vi "S2C_SetXmlOutput.vi"(8 "Error In":errorcluster, 11 "MenuRef":refnum<k9>) -> (0 "Error Out":errorcluster)   [LabVIEW 2015]
doc: "Toggles the \"Local File\" runtime menu item."
uses:
  XML/S2C_XML_Globals.vi
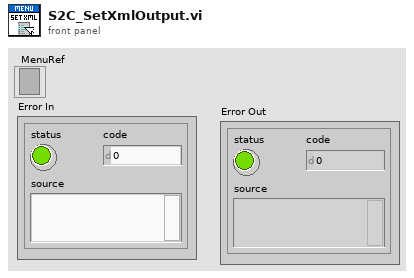
[diagram p1: front panel]
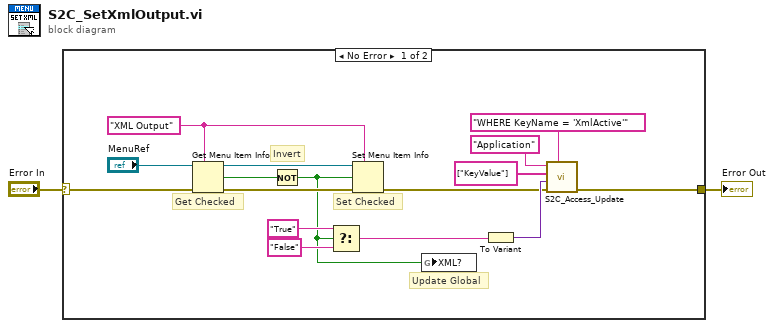
[diagram p0: block diagram]
diagram:
  n1 = case shown="No Error" "Error In" {
    selector: "Error In" -> [w18 w19]
    tunnel: [w5 w19] -> w1
    frame No Error {
      w16 = "XML Output" ("item tag")
      # "Update Global"
      # "Invert"
      # "Set Checked"
      # "Get Checked"
      n2 = Get Menu Item Info(7:w16, 8:w18, 11:"MenuRef") -> (0:w15:errorcluster, 3:w14:refnum<k9>, 4:w13:bool)  [unwired: 4 out]
      n3 = Not(x=w13) -> (.not. x?=w3:bool)
      n4 = Select(t="True", s=w3, f="False") -> (s? t:f=w4:string)
      n5 = Set Menu Item Info(6:w3, 7:w16, 8:w15, 11:w14) -> (0:w6:errorcluster)  [unwired: 3 in, 1 out]
      n6 = global write "S2C_XML_Globals.vi" "XML?"(w3) -> ()
      n7 = To Variant(anything=w4) -> (Variant=w8:variant)
      n8 = call "S2C_Access_Update.vi"("Condition"="WHERE KeyName = 'XmlActive'", "Error In"=w6, "Data"=w8, "Columns"=string[] ["KeyValue"], "Table"="Application") -> ("Error Out"=w5:errorcluster)  [unwired: 6 in]
    }
    frame Error {
    }
  }
  "Error Out" <- w1
